vi "Format table.vi"(11 "Table输入":refnum<vi>) -> ()   [LabVIEW 2016, in "main.lvlib"]
uses:
  main.lvlib
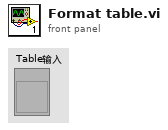
[diagram p1: front panel]
types:
  T1 = cluster{"Font Name:":string, "Size":i16, "Strikeout?":bool, "Italic?":bool, "Underline?":bool, "Outline?":bool, "Shadow?":bool, "Bold?":bool}
  T2 = typedef "LVFontTypeDef.ctl" = cluster{"Font Name":string, "Size":u16, "Bold":bool, "Italic":bool, "Underline":bool, "Strikeout":bool, "Color":u32}
  T3 = enum16{"User-specified Font", "Application Font", "System Font", "Dialog Font"}
  T4 = cluster{"left":i16, "top":i16, "right":i16, "bottom":i16}
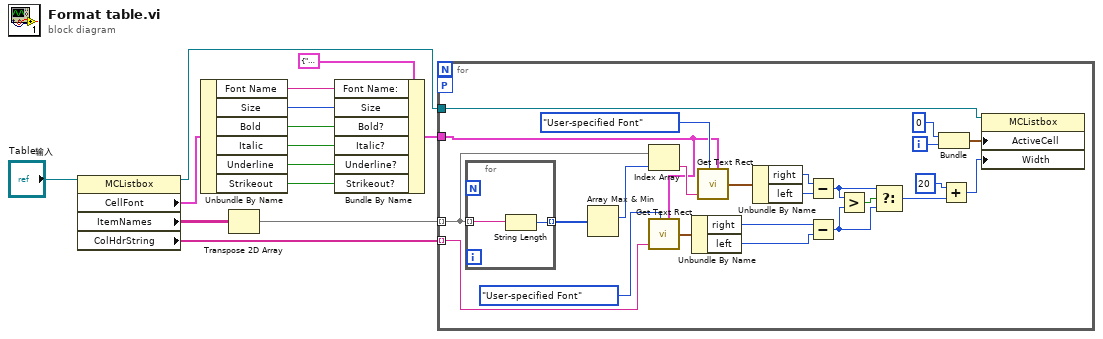
[diagram p0: block diagram]
diagram:
  n1 = property class="MCListbox"(reference="Table输入") -> (reference out=w1:refnum<vi>, "CellFont"=w5:T2, "ItemNames"=w14:string[][], "ColHdrString"=w2:string[])  [unwired: 1 in, 1 out]
  n2 = Unbundle By Name(w5) -> ("Font Name"=w11:string, "Size"=w10:u16, "Bold"=w9:bool, "Italic"=w8:bool, "Underline"=w7:bool, "Strikeout"=w6:bool)
  n3 = Transpose 2D Array(2D array=w14) -> (transposed array=w13:string[][])
  n4 = Bundle By Name(cluster=T1 {"Font Name:"="", "Size"=0, "Strikeout?"=FALSE, "Italic?"=FALSE, "Underline?"=FALSE, "Outline?"=FALSE, "Shadow?"=FALSE, "Bold?"=FALSE} ("[user-specified font]"), "Font Name:"=w11, "Size"=w10, "Bold?"=w9, "Italic?"=w8, "Underline?"=w7, "Strikeout?"=w6) -> (w3:T1)
  n5 = for {
    tunnel: w13 -> [w20] mode=indexing
    tunnel: w1 -> [w16]
    tunnel: w2 -> [w28] mode=indexing
    workers-P: _ -> [_]
    tunnel: w3 -> [w17]
    i -> [w38]
    n6 = for {
      tunnel: w20 -> [w40] mode=indexing
      tunnel: [w39] -> w19 mode=indexing
      n7 = String Length(string=w40) -> (length=w39:i32)
    }
    n8 = Array Max & Min(array=w19) -> (max index (indices)=w18:i32)  [unwired: 3 out]
    n9 = Index Array(array=w20, index=w18) -> (element=w30:string)
    n10 = call <vilib>:"Get Text Rect.vi"("desired font(Application)"=T3."User-specified Font", "text"=w28, "[user-specified font]"=w17) -> ("rect"=w25:T4)  [unwired: 6 in]
    n11 = Unbundle By Name(w25) -> ("right"=w26:i16, "left"=w27:i16)
    n12 = call <vilib>:"Get Text Rect.vi"("desired font(Application)"=T3."User-specified Font", "text"=w30, "[user-specified font]"=w17) -> ("rect"=w33:T4)  [unwired: 6 in]
    n13 = Unbundle By Name(w33) -> ("right"=w32:i16, "left"=w31:i16)
    n14 = Subtract(x=w32, y=w31) -> (x-y=w23:i16)
    n15 = Subtract(x=w26, y=w27) -> (x-y=w22:i16)
    n16 = Greater?(x=w23, y=w22) -> (0:w24:bool)
    n17 = Select(t=w23, s=w24, f=w22) -> (s? t:f=w21:i16)
    n18 = Bundle(0, w38) -> (w15:cluster{i32, i32})  [unwired: 1 in]
    n19 = Add(x=i16 20, y=w21) -> (x+y=w35:i16)
    n20 = property on="属性节点" class="MCListbox"(reference=w16, "ActiveCell"=w15, "Width"=w35) -> ()  [unwired: 1 in, 2 out]
  }
